vi "Drive Simple.vi"(10 "Data":string[](array[string]), 11 "Robot dev revs":T1) -> (3 "Robot dev revs out":T1)   [LabVIEW 2013]
uses:
  Robot dev revs.ctl
  Drive typedef.ctl
  Drive Motors Typedef.ctl
  GearBox Typedef.ctl
  <vilib>/Rock Robotics/WPI/MotorControl/WPI_MotorControlDeviceRef.ctl
  <vilib>/Rock Robotics/SystemInterfaces/Typedef/FPGA_TypedefDigitalModule.ctl
  <vilib>/Rock Robotics/SystemInterfaces/DIO/FPGA_DIOPWMChannel.ctl
  <vilib>/Rock Robotics/WPI/PWM/WPI_PWMDeadband.ctl
  <vilib>/Rock Robotics/WPI/CAN/Jaguar/SubVIs/WPI_CANJaguar_ControlMode.ctl
  <vilib>/Rock Robotics/WPI/PWM/WPI_PWMTransform_ConPane.ctl
  <vilib>/Rock Robotics/WPI/Solenoid/WPI_SolenoidDevRef.ctl
  <vilib>/Rock Robotics/SystemInterfaces/Typedef/FPGA_TypedefSolenoidModule.ctl
  <vilib>/Rock Robotics/WPI/Solenoid/WPI_SolenoidChannel.ctl
  Drive Sensor Typedef.ctl
  <vilib>/Rock Robotics/WPI/Encoder/WPI_EncoderDevRef.ctl
  <vilib>/Rock Robotics/SystemInterfaces/Encoder/FPGA_EncoderIdx.ctl
  <vilib>/Rock Robotics/SystemInterfaces/Counter/FPGA_CounterCtrSystemIndex.ctl
  <vilib>/Rock Robotics/WPI/Encoder/WPI_EncoderType.ctl
  <vilib>/Rock Robotics/WPI/Gyro/WPI_GyroDevRef.ctl
  <vilib>/Rock Robotics/SystemInterfaces/Typedef/FPGA_TypedefAnalogModule.ctl
  <vilib>/Rock Robotics/SystemInterfaces/AI/FPGA_AIChannel.ctl
  catapult code/catapult type def.ctl
  <vilib>/Rock Robotics/WPI/DigitalInput/WPI_DigitalInputDevRef.ctl
  <vilib>/Rock Robotics/SystemInterfaces/DIO/FPGA_DIOChannel.ctl
  <vilib>/Rock Robotics/WPI/Joystick/WPI_JoystickDevRef.ctl
  <vilib>/Rock Robotics/WPI/Joystick/WPI_JoystickDeviceEnum.ctl
  Roller V2/roller typedef.ctl
  Puncher/Puncher type.ctl
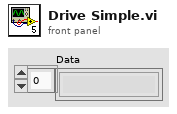
[diagram p1: front panel]
types:
  T1 = typedef "Robot dev revs.ctl" = cluster{"Drive":T2, "Catapult devrevs":T23, "Drive Joystick":T26, "Operator Joystick":T26, "roller devrevs":T28, "Puncher devrevs":T29}
  T2 = typedef "Drive typedef.ctl" = cluster{"Drive Actuaters":cluster{"Motor devRevs":T3, "SolenoidDevRef":T12}, "Drive Sensor data":T15}
  T3 = typedef "Drive Motors Typedef.ctl" = cluster{"Left Side Motors":T4, "Right Side Motors":T4, "dev Status":errorcluster}
  T4 = typedef "GearBox Typedef.ctl" = cluster{"Motor 1 devRev":T5, "Motor 2 devRev":T5, "Motor 3 devRev":T5}
  T5 = typedef "WPI_MotorControlDeviceRef.ctl" = cluster{"DeviceStatus":errorcluster, "Type":enum16{"PWM", "CAN"}, "PWM":cluster{"Digital Module":T6, "PWM Channel":T7, "DeadBand":T8}, "CAN":cluster{"Device Number":u8, "Control Mode":T9, "Semaphore":T10, "Max Vout":dbl}, "Invert":bool, "TransformRef":T11, "InvTransformRef":T11}
  T6 = typedef "FPGA_TypedefDigitalModule.ctl" = enum16{"Digital Module 1", "Digital Module 2"}
  T7 = typedef "FPGA_DIOPWMChannel.ctl" = enum8{"PWM 1", "PWM 2", "PWM 3", "PWM 4", "PWM 5", "PWM 6", "PWM 7", "PWM 8", "PWM 9", "PWM 10", "Invalid"}
  T8 = typedef "WPI_PWMDeadband.ctl" = cluster{"Name":string, "maxPositivePwm":i32, "minPositivePwm":i32, "centerPwm":i32, "maxNegativePwm":i32, "minNegativePwm":i32, "angularRange":u16}
  T9 = typedef "WPI_CANJaguar_ControlMode.ctl" = enum8{"Percent VBus", "Current", "Speed", "Position", "Voltage"}
  T10 = typedef "Semaphore RefNum" = refnum<k1>
  T11 = typedef "WPI_PWMTransform_ConPane.ctl" = refnum<vi>
  T12 = typedef "WPI_SolenoidDevRef.ctl" = cluster{"DevStatus":errorcluster, "Solenoid Module":T13, "Forward Solenoid Channel":T14, "Reverse Solenoid Channel":T14}
  T13 = typedef "FPGA_TypedefSolenoidModule.ctl" = enum16{"Solenoid Module 1", "Solenoid Module 2"}
  T14 = typedef "WPI_SolenoidChannel.ctl" = enum8{"Solenoid 1", "Solenoid 2", "Solenoid 3", "Solenoid 4", "Solenoid 5", "Solenoid 6", "Solenoid 7", "Solenoid 8", "Invalid"}
  T15 = typedef "Drive Sensor Typedef.ctl" = cluster{"Encoders":cluster{"Right Encoder":T16}, "GyroDevRef":T20, "Last commanded Angle":dbl}
  T16 = typedef "WPI_EncoderDevRef.ctl" = cluster{"DevStatus":errorcluster, "EncoderIndex":T17, "CounterIndex":T18, "DistancePerCount":dbl, "Decoding Type":T19}
  T17 = typedef "FPGA_EncoderIdx.ctl" = enum8{"Enc 0", "Enc 1", "Enc 2", "Enc 3", "Invalid"}
  T18 = typedef "FPGA_CounterCtrSystemIndex.ctl" = enum8{"Ctr 0", "Ctr 1", "Ctr 2", "Ctr 3", "Ctr 4", "Ctr 5", "Ctr 6", "Ctr 7", "Invalid"}
  T19 = typedef "WPI_EncoderType.ctl" = enum16{"1x", "2x", "4x"}
  T20 = typedef "WPI_GyroDevRef.ctl" = cluster{"DevStatus":errorcluster, "Analog Module":T21, "Analog Channel":T22, "Offset":dbl, "Gain (VoltsPerDegree/Second)":dbl}
  T21 = typedef "FPGA_TypedefAnalogModule.ctl" = enum16{"Analog Module 1", "Analog Module 2"}
  T22 = typedef "FPGA_AIChannel.ctl" = enum8{"AI 1", "AI 2", "AI 3", "AI 4", "AI 5", "AI 6", "AI 7", "AI 8", "Invalid"}
  T23 = typedef "catapult type def.ctl" = cluster{"MotorControlDeviceRef":T5, "SolenoidDevRef":T12, "first limit switch":T24, "second limit switch":T24}
  T24 = typedef "WPI_DigitalInputDevRef.ctl" = cluster{"DevStatus":errorcluster, "DIO Channel":T25, "Digital Module":T6}
  T25 = typedef "FPGA_DIOChannel.ctl" = enum8{"DIO 1", "DIO 2", "DIO 3", "DIO 4", "DIO 5", "DIO 6", "DIO 7", "DIO 8", "DIO 9", "DIO 10", "DIO 11", "DIO 12", "DIO 13", "DIO 14", "Invalid"}
  T26 = typedef "WPI_JoystickDevRef.ctl" = cluster{"Device":T27}
  T27 = typedef "WPI_JoystickDeviceEnum.ctl" = enum16{"USB 1", "USB 2", "USB 3", "USB 4", "Kinect 1", "Kinect 2"}
  T28 = typedef "roller typedef.ctl" = cluster{"SolenoidDevRef":T12, "MotorControlDeviceRef":T5, "DigitalInputDevRef":T24}
  T29 = typedef "Puncher type.ctl" = cluster{"SolenoidDevRef":T12, "DigitalInputDevRef":T24}
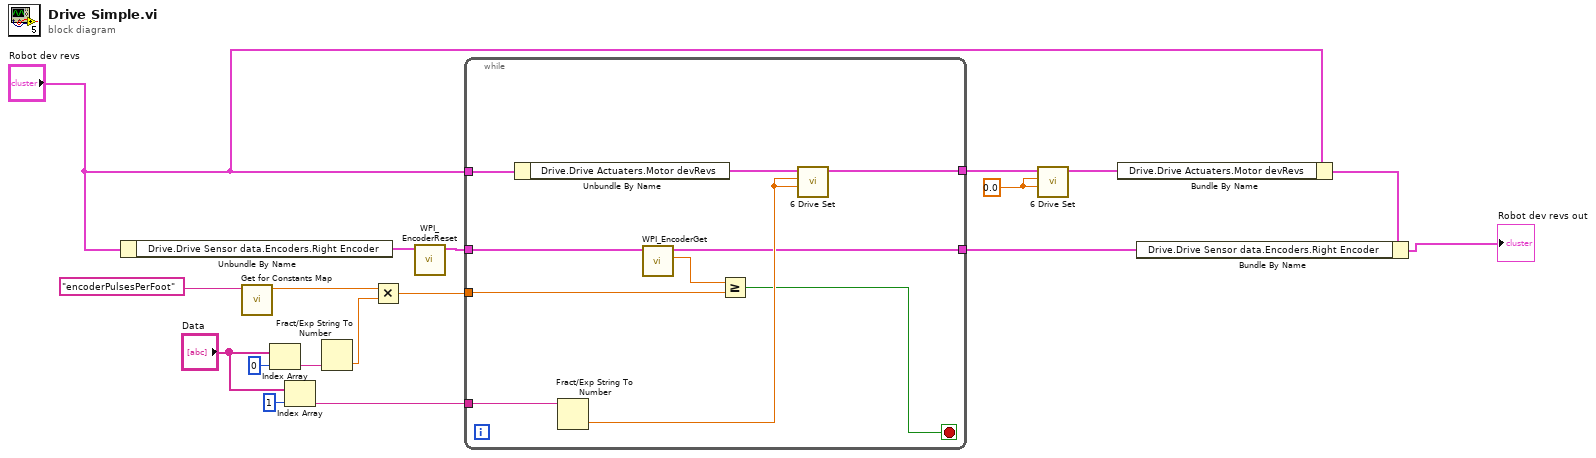
[diagram p0: block diagram]
diagram:
  w9 = 0.0 ("Left side speed")
  n1 = Unbundle By Name("Robot dev revs") -> ("Drive.Drive Sensor data.Encoders.Right Encoder"=w6:T16)
  n2 = call "Get for Constants Map.vi"("Constant Name"="encoderPulsesPerFoot") -> ("Value"=w14:dbl)  [unwired: 8 in, 2 out]
  n3 = Index Array(array="Data", index=0) -> (element=w12:string)
  n4 = Index Array(array="Data", index=1) -> (element=w13:string)
  n5 = Fract/Exp String To Number(string=w12) -> (number=w11:dbl)  [unwired: 3 in, 1 out]
  n6 = Multiply(x=w14, y=w11) -> (x*y=w10:dbl)
  n7 = call <vilib>:"WPI_EncoderReset.vi"("EncoderDevRef"=w6) -> ("EncoderDevRef"=w7:T16)  [unwired: 9 in, 1 out]
  n8 = while {
    tunnel: "Robot dev revs" -> [w25]
    tunnel: w13 -> [w28]
    tunnel: w10 -> [w23]
    tunnel: [w21] -> w8
    tunnel: w7 -> [w20]
    tunnel: [w19] -> w2
    stop <- w22 stop-if-true
    n9 = Unbundle By Name(w25) -> ("Drive.Drive Actuaters.Motor devRevs"=w26:T3)
    n10 = Fract/Exp String To Number(string=w28) -> (number=w27:dbl)  [unwired: 3 in, 1 out]
    n11 = call <vilib>:"WPI_EncoderGet.vi"("EncoderDevRef"=w20) -> ("Distance"=w24:dbl, "EncoderDevRef"=w19:T16)  [unwired: 5 in, 4 out]
    n12 = Greater Or Equal?(x=w24, y=w23) -> (x >= y?=w22:bool)
    n13 = call "6 Drive Set.vi"("Motor devRevs"=w26, "Left side speed"=w27, "Right side speed"=w27) -> ("Motor devRevs"=w21:T3)  [unwired: 6 in, 1 out]
  }
  n14 = call "6 Drive Set.vi"("Motor devRevs"=w8, "Left side speed"=w9, "Right side speed"=w9) -> ("Motor devRevs"=w3:T3)  [unwired: 6 in, 1 out]
  n15 = Bundle By Name(cluster="Robot dev revs", "Drive.Drive Actuaters.Motor devRevs"=w3) -> (w4:T1)
  n16 = Bundle By Name(cluster=w4, "Drive.Drive Sensor data.Encoders.Right Encoder"=w2) -> (→"Robot dev revs out":T1)
